vi "Tenerowicz_Target_C_1.vi"   [LabVIEW 2023]
uses:
  <vilib>/Platform/TimedLoop/XDataNode/timing_clust.ctl
  <vilib>/Platform/TimedLoop/XDataNode/nitl_modes.ctl
  <vilib>/Platform/TimedLoop/XDataNode/wakeup.ctl
  <vilib>/platform/TimedLoop/XDataNode/XDataNode.xnode
  <vilib>/Platform/TimedLoop/XDataNode/XDNodeRunTimeDep.lvlib
types:
  T1 = typedef "XDNodeRunTimeDep.lvlib/timing_clust.ctl" = cluster{"Expected End [f-1]":u64, "Actual End [f-1]":u64, "Finished Late? [f-1]":bool, "Expected End [i-1]":u64, "Actual End [i-1]":u64, "Finished Late? [i-1]":bool, "Expected Start [i]":u64, "Actual Start [i]":u64, "Expected Start [f]":u64, "Actual Start [f]":u64, "Source Name":string, "Structure Name":string, "Period":i64, "Deadline":i64, "Offset":i64, "Start":i64, "Priority":i32, "Timeout":i32, "Mode":T2, "Wakeup Reason":T3, "Error":errorcluster, "Source Type":string, "Secondary Source Type":string, "Global End Time":u64, "Global Start Time":u64, "Frame Duration":u64, "Iteration Duration":u64, "Assigned CPU":i32, "I/O Scan Engine Mode":u32}
  T2 = typedef "XDNodeRunTimeDep.lvlib/nitl_modes.ctl" = enum32{"No Change", "Process missed periods, maintain original phase", "Discard missed periods, maintain original phase", "Process missed periods, ignore original phase", "Discard missed periods, ignore original phase"}
  T3 = typedef "XDNodeRunTimeDep.lvlib/wakeup.ctl" = enum32{"Normal", "Aborted", "Asynchronous wakeup", "Timing source error", "Timed loop error", "Timeout"}
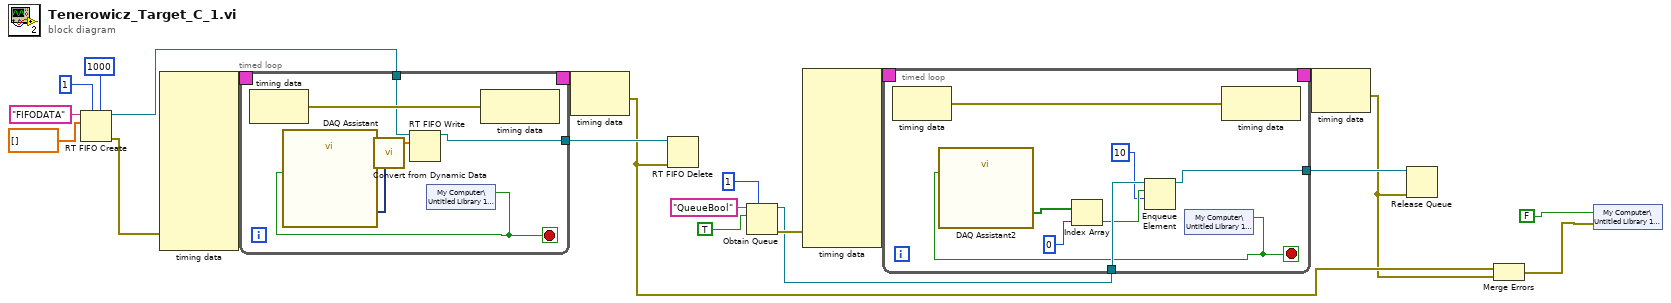
[diagram p0: block diagram]
diagram:
  n1 = RT FIFO Create(0:"FIFODATA" ("name (unnamed)"), 1:dbl[] [] ("type"), 4:u32 1 ("size (10)"), 6:u32 1000 ("elements in array (1)")) -> (8:w12:refnum<k33>, 11:w17:errorcluster)  [unwired: 4 in, 1 out]
  n2 = node-c288(w17) -> (w21:T1)  [unwired: 9 in]
  n3 = timed-loop {
    timing: w21 -> [_]
    timing-out: [_] -> w20
    tunnel: w12 -> [w26]
    tunnel: [w23] -> w11
    stop <- w22 stop-if-true
    n4 = node-c288() -> (w27:errorcluster)  [unwired: 1 in]
    n5 = shared-variable "My Computer\\Untitled Library 1.lvlib\\Stop"() -> (w22:bool)  [unwired: 1 in, 1 out]
    n6 = call "DAQ Assistant"("stop (T)"=w22) -> ("data"=w25:dynamicdata)  [unwired: 16 in, 2 out]
    n7 = call "Convert from Dynamic Data"("Dynamic Data Type"=w25) -> ("Array"=w24:dbl[])  [unwired: 3 in]
    n8 = RT FIFO Write(0:w26, 1:w24) -> (8:w23:refnum<k33>)  [unwired: 3 in, 3 out]
    n9 = node-c288(w27) -> ()  [unwired: 1 out]
  }
  n10 = node-c288(w20) -> (w4:errorcluster)
  n11 = RT FIFO Delete(0:w11, 3:w4) -> ()  [unwired: 1 in, 1 out]
  n12 = Obtain Queue(max queue size (-1, unlimited)=1, name (unnamed)="QueueBool", element data type=TRUE) -> (queue out=w6:refnum<queue>, error out=w7:errorcluster)  [unwired: 2 in, 1 out]
  n13 = node-c288(w7) -> (w19:T1)  [unwired: 9 in]
  n14 = timed-loop {
    timing: w19 -> [_]
    timing-out: [_] -> w18
    tunnel: w6 -> [w39]
    tunnel: [w35] -> w5
    stop <- w33 stop-if-true
    n15 = node-c288() -> (w40:errorcluster)  [unwired: 1 in]
    n16 = shared-variable "My Computer\\Untitled Library 1.lvlib\\Stop"() -> (w33:bool)  [unwired: 1 in, 1 out]
    n17 = call "DAQ Assistant2"("stop (T)"=w33) -> ("data"=w36:bool[])  [unwired: 16 in, 2 out]
    n18 = Index Array(array=w36, index=0) -> (element=w37:bool)
    n19 = Enqueue Element(queue=w39, element=w37, timeout in ms (-1)=10) -> (queue out=w35:refnum<queue>)  [unwired: 1 in, 2 out]
    n20 = node-c288(w40) -> ()  [unwired: 1 out]
  }
  n21 = node-c288(w18) -> (w3:errorcluster)
  n22 = Release Queue(queue=w5, error in (no error)=w3) -> ()  [unwired: 1 in, 3 out]
  n23 = Merge Errors(w4, w3) -> (w2:errorcluster)
  n24 = shared-variable "My Computer\\Untitled Library 1.lvlib\\Stop"(FALSE, error in=w2) -> ()  [unwired: 1 out]
